vi "SetHistDataName.vi"(7 "ForceSet":bool, 8 "error in (no error)":errorcluster caption="entrée d'erreur (pas d'erreur)", 9 "SetInpChan":T1[](array[typedef]), 10 "Channels":T3[](array[typedef]) {"DeadTime" min=800 max=160000 step=1; "Edge" items=["falling", "rising"]; "Offset" min=-100000 max=100000 step=5; "Level" min=-1200 max=1200 step=1}, 11 "MultiHarp150.lvclass":refnum<class "MultiHarp150.lvclass">) -> (0 "error out":errorcluster caption="sortie d'erreur", 3 "MultiHarp150.lvclass Out":refnum<class "MultiHarp150.lvclass">)   [LabVIEW 2019, in "MultiHarp150.lvclass"]
uses:
  MultiHarp150.lvclass
  C:/Programmes Labview/LabScanV1A/DevicesClass/BaseDevice/BaseDevice.lvclass
  <userlib>/MultiHarp150/MH_InputChannel_LS.ctl
  <userlib>/MultiHarp150/UIThread/MH_SetInpChanData.ctl
  <userlib>/MultiHarp150/UIThread/MH_SetInpChanCmds.ctl
  MultiHarp150.lvclass/MultiHarp150.ctl
  BaseDevice/BaseDevice.lvclass/BaseDevice.ctl
  BaseDevice/Accessor/SetShowInstrNm.vi
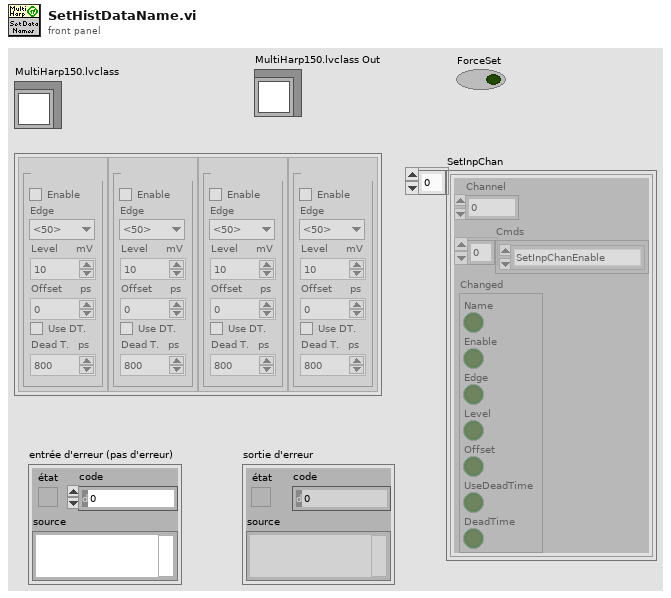
[diagram p1: front panel]
types:
  T1 = typedef "MH_SetInpChanData.ctl" = cluster{"Channel":i32, "Cmds":T2[], "Changed":cluster{"Name":bool, "Enable":bool, "Edge":bool, "Level":bool, "Offset":bool, "UseDeadTime":bool, "DeadTime":bool}}
  T2 = typedef "MH_SetInpChanCmds.ctl" = enum16{"SetInpChanEnable", "SetInpChanOffset", "SetInpChanDeadTime", "SetInpChanTrg"}
  T3 = typedef "MH_InputChannel_LS.ctl" = cluster{"Name":string, "Enable":bool, "Edge":i32, "Level":i32, "Offset":i32, "UseDeadTime":bool, "DeadTime":i32}
  T4 = typedef "MultiHarp150.lvclass/MultiHarp150_Func.ctl" = enum16{"ReadHistogram (Ph)", "ReadT2 (Ph)", "ReadT3 (Ph)", "ReadCount (Ph)"}
  T5 = typedef "MH_MeasMode.ctl" = i32
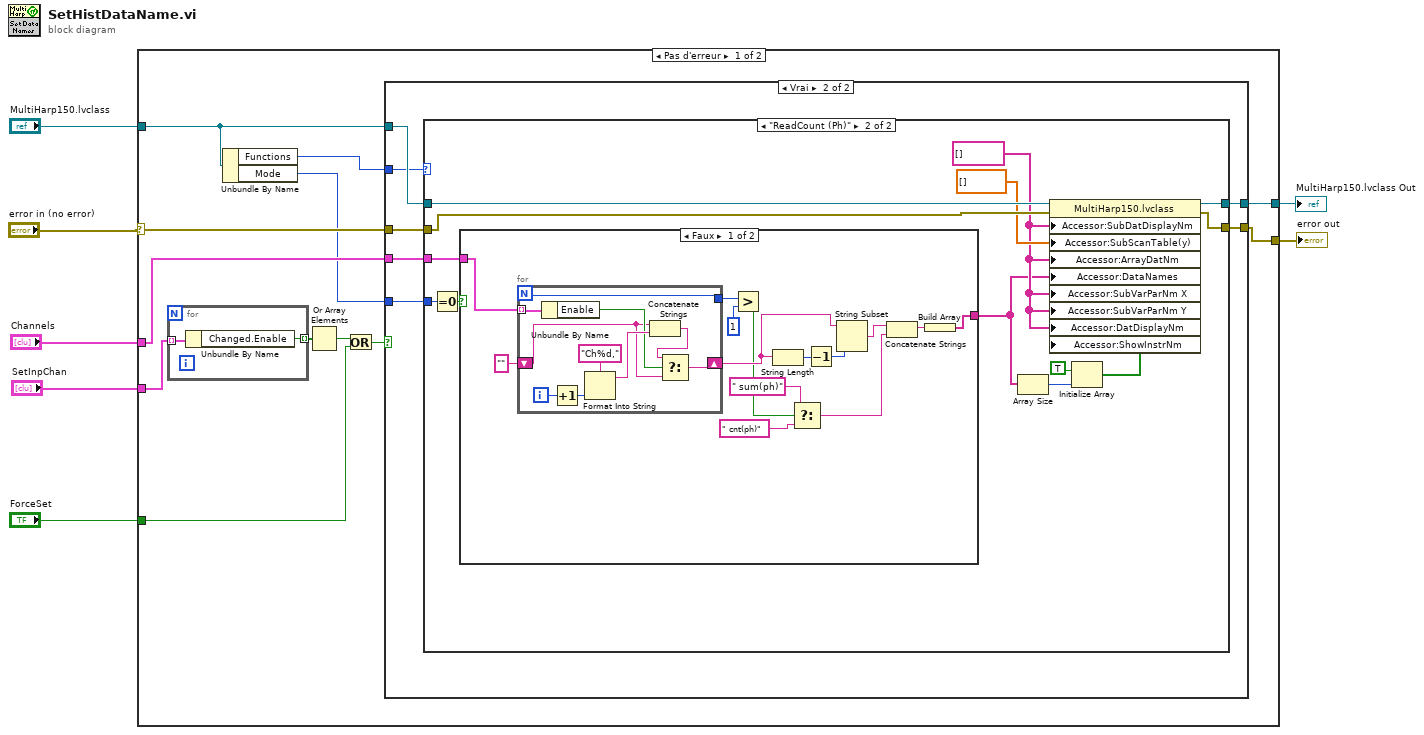
[diagram p0: block diagram]
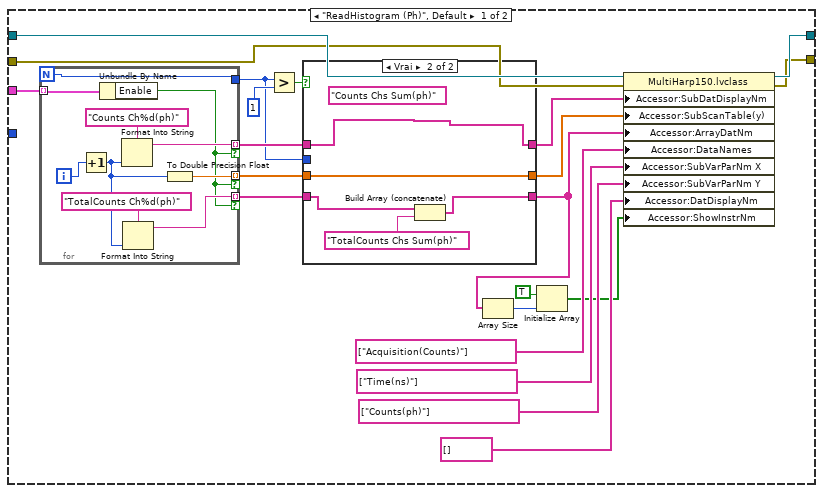
[diagram p3: hidden frame]
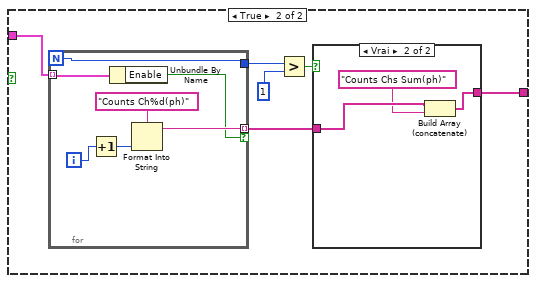
[diagram p5: hidden frame]
diagram:
  n1 = case shown="Pas d'erreur" "error in (no error)" {
    selector: "error in (no error)" -> [w19 w124]
    tunnel: "MultiHarp150.lvclass" -> [w10 w125]
    tunnel: "Channels" -> [w17 _]
    tunnel: [w16 w125] -> w4
    tunnel: [w15 w124] -> w3
    tunnel: "SetInpChan" -> [w14 _]
    tunnel: "ForceSet" -> [w11 _]
    frame No Error {
      n2 = for {
        tunnel: w14 -> [w21] mode=indexing
        tunnel: [w20] -> w18 mode=indexing
        n3 = Unbundle By Name(w21) -> ("Changed.Enable"=w20:bool)
      }
      n4 = Unbundle By Name(w10) -> ("Functions"=w9:T4, "Mode"=w8:T5)
      n5 = Or Array Elements(Boolean array=w18) -> (logical OR=w12:bool)
      n6 = Or(x=w12, y=w11) -> (x .or. y?=w13:bool)
      n7 = case shown="Vrai" w13 {
        tunnel: w10 -> [w23 w30]
        tunnel: [w23 w29] -> w16
        tunnel: w17 -> [_ w28]
        tunnel: [w22 w27] -> w15
        tunnel: w19 -> [w22 w26]
        tunnel: w9 -> [_ w25]
        tunnel: w8 -> [_ w24]
        frame False {
        }
        frame True {
          n8 = case shown="\"ReadCount (Ph)\"" w25 {
            tunnel: w30 -> [w51 w82]
            tunnel: [w50 w81] -> w29
            tunnel: w28 -> [w49 w80]
            tunnel: [w48 w79] -> w27
            tunnel: w26 -> [w47 w78]
            tunnel: w24 -> [_ w71]
            frame "ReadHistogram (Ph)", Default {
              n9 = for {
                N -> [w61]
                tunnel: w49 -> [w69] mode=indexing
                tunnel: [w66] -> w41 mode=indexing if=w62
                tunnel: [w65] -> w45 mode=indexing if=w62
                tunnel: [w63] -> w43 mode=indexing if=w62
                tunnel: [w61] -> w39
                i -> [w68]
                n10 = Increment(x=w68) -> (x+1=w64:i32)
                n11 = Unbundle By Name(w69) -> ("Enable"=w62:bool)
                n12 = Format Into String(format string="Counts Ch%d(ph)" ("chaîne de format"), w64) -> (resulting string=w66:string)  [unwired: 2 in, 1 out]
                n13 = Format Into String(format string="TotalCounts Ch%d(ph)" ("chaîne de format"), w64) -> (resulting string=w65:string)  [unwired: 2 in, 1 out]
                n14 = To Double Precision Float(number=w64) -> (double precision float=w63:dbl)
              }
              n15 = Greater?(x=w39, y=1) -> (0:w40:bool)
              n16 = case shown="Vrai" w40 {
                tunnel: [w54 w57] -> w32
                tunnel: w45 -> [w54 w59]
                tunnel: [w53 w55] -> w44
                tunnel: w43 -> [w53 w55]
                tunnel: [w52 w56] -> w42
                tunnel: w41 -> [w52 w56]
                tunnel: w39 -> [_ _]
                frame False {
                }
                frame True {
                  (unwired) "Counts Chs Sum(ph)" ("chaîne de format")
                  n17 = Build Array (concatenate)(w59, "TotalCounts Chs Sum(ph)" ("chaîne de format")) -> (w57:string[])
                }
              }
              n18 = Array Size(array=w32) -> (size(s)=w34:i32)
              n19 = Initialize Array(TRUE, w34) -> (w31:bool[])
              n20 = property class="MultiHarp150.lvclass"(reference=w51, error in=w47, "Accessor:SubDatDisplayNm"=w42, "Accessor:SubScanTable(y)"=w44, "Accessor:ArrayDatNm"=w32, "Accessor:DataNames"=string[] ["Acquisition(Counts)"], "Accessor:SubVarParNm X"=string[] ["Time(ns)"], "Accessor:SubVarParNm Y"=string[] ["Counts(ph)"], "Accessor:DatDisplayNm"=string[] [] ("DatDisplayNm"), "Accessor:ShowInstrNm"=w31) -> (reference out=w50:refnum<class "MultiHarp150.lvclass">, error out=w48:errorcluster)
            }
            frame "ReadCount (Ph)" {
              w76 = string[] []
              n21 = Equal To 0?(x=w71) -> (x = 0?=w70:bool)
              n22 = case shown="Faux" w70 {
                tunnel: w80 -> [w84 w112]
                tunnel: [w83 w107] -> w73
                frame False {
                  n23 = for {
                    N -> [w102]
                    tunnel: w84 -> [w106] mode=indexing
                    tunnel: [w102] -> w95
                    shift-right: [w97] -> w90
                    shift-left: "" -> [w98]
                    i -> [w105]
                    n24 = Unbundle By Name(w106) -> ("Enable"=w99:bool)
                    n25 = Increment(x=w105) -> (x+1=w103:i32)
                    n26 = Format Into String(format string="Ch%d," ("chaîne de format"), w103) -> (resulting string=w101:string)  [unwired: 2 in, 1 out]
                    n27 = Concatenate Strings(w98, w101) -> (w100:string)
                    n28 = Select(t=w100, s=w99, f=w98) -> (s? t:f=w97:string)
                  }
                  n29 = Greater?(x=w95, y=1) -> (0:w88:bool)
                  n30 = String Length(string=w90) -> (length=w92:i32)
                  n31 = Select(t=" sum(ph)" ("chaîne"), s=w88, f=" cnt(ph)" ("chaîne")) -> (s? t:f=w85:string)
                  n32 = Decrement(x=w92) -> (x-1=w91:i32)
                  n33 = String Subset(string=w90, length (rest)=w91) -> (substring=w89:string)  [unwired: 1 in]
                  n34 = Concatenate Strings(w89, w85) -> (w94:string)
                  n35 = Build Array(w94) -> (w83:string[])
                }
                frame True {
                  n36 = for {
                    N -> [w117]
                    tunnel: w112 -> [w123] mode=indexing
                    tunnel: [w120] -> w110 mode=indexing if=w118
                    tunnel: [w117] -> w108
                    i -> [w122]
                    n37 = Increment(x=w122) -> (x+1=w119:i32)
                    n38 = Unbundle By Name(w123) -> ("Enable"=w118:bool)
                    n39 = Format Into String(format string="Counts Ch%d(ph)" ("chaîne de format"), w119) -> (resulting string=w120:string)  [unwired: 2 in, 1 out]
                  }
                  n40 = Greater?(x=w108, y=1) -> (0:w109:bool)
                  n41 = case shown="Vrai" w109 {
                    tunnel: w110 -> [w113 w116]
                    tunnel: [w113 w114] -> w107
                    frame False {
                    }
                    frame True {
                      n42 = Build Array (concatenate)(w116, "Counts Chs Sum(ph)" ("chaîne de format")) -> (w114:string[])
                    }
                  }
                }
              }
              n43 = Array Size(array=w73) -> (size(s)=w75:i32)
              n44 = Initialize Array(TRUE, w75) -> (w72:bool[])
              n45 = property class="MultiHarp150.lvclass"(reference=w82, error in=w78, "Accessor:SubDatDisplayNm"=w76, "Accessor:SubScanTable(y)"=dbl[] [], "Accessor:ArrayDatNm"=w76, "Accessor:DataNames"=w73, "Accessor:SubVarParNm X"=w76, "Accessor:SubVarParNm Y"=w76, "Accessor:DatDisplayNm"=w76, "Accessor:ShowInstrNm"=w72) -> (reference out=w81:refnum<class "MultiHarp150.lvclass">, error out=w79:errorcluster)
            }
          }
        }
      }
    }
    frame Error {
    }
  }
  "error out" <- w3
  "MultiHarp150.lvclass Out" <- w4
